vi "ex5-2.vi"   [LabVIEW 2014]
uses:
  <vilib>/NXT/Subs/MotorOutput.ctl
  <vilib>/NXT/Dual Mode Library/Motors/MotorOn.vi
  <vilib>/NXT/Dual Mode Library/Waits/Wait_Num.vi
  <vilib>/NXT/Dual Mode Library/Motors/MotorBrake.vi
types:
  T1 = typedef "MotorOutput.ctl" = u8
  T2 = typedef "LVHSConnector.ctl" = refnum<class "BrickReference.lvclass">
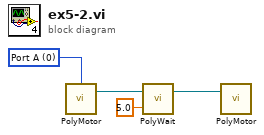
[diagram p0: block diagram]
diagram:
  w1 = T1 0 items=["Port A"=0, "Port B"=1, "Port C"=2, "Ports A & B"=4, "Ports A & C"=5, "Ports B & C"=6, "All Ports"=3] ("Output Port (All Ports)")
  n1 = call-poly <vilib>:"PolyMotor.vi"("Output Port (All Ports)"=w1) -> ("NXT/EV3"=w4:T2)  [unwired: 3 in]
  n2 = call-poly <vilib>:"PolyWait.vi"("Time (1 sec)"=sgl 5.0, "NXT/EV3"=w4) -> ("NXT/EV3"=w3:T2)  [unwired: 2 in]
  n3 = call-poly <vilib>:"PolyMotor.vi"("NXT/EV3"=w3) -> ()  [unwired: 3 in, 1 out]
